vi "Update Ctrls.vi"(8 "error in (no error)":errorcluster, 10 "Columns (All)":string[](array[string]), 11 "Basic Form in":refnum<class "Basic Form.lvclass">) -> (0 "error out":errorcluster, 3 "Basic Form out":refnum<class "Basic Form.lvclass">)   [LabVIEW 2020, in "Form.lvlib" / "Basic Form.lvclass"]
uses:
  Basic Form.lvclass
  C:/Users/User/Desktop/Raman Program/Database OOP/source/Database OOP/Table Libraries/Basic Table/Basic Table Class/Basic Table.lvclass
  Basic Table/Basic Table Class/Basic Table.lvclass/Basic Table.ctl
  Basic Form.lvclass/Basic Form.ctl
  Column Libraries/Field Interfaces/Field Interface Class/Field Interface.lvclass
  C:/Users/User/Desktop/Raman Program/Database OOP/source/Database OOP/Column Libraries/Column Interface/Column Interface Class/Column Interface.lvclass
  Column Libraries/Column Interface/Column Interface Class/Column Interface.lvclass
  Basic Table/Basic Table Class/Basic Table.lvclass
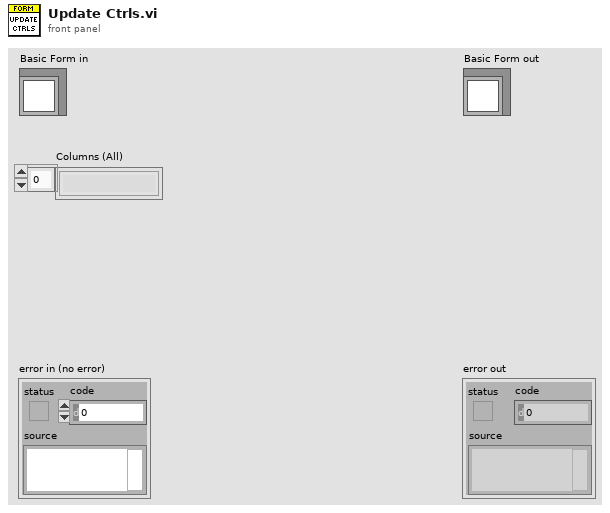
[diagram p1: front panel]
types:
  T1 = map{string, refnum<class "Column Interface.lvclass">}
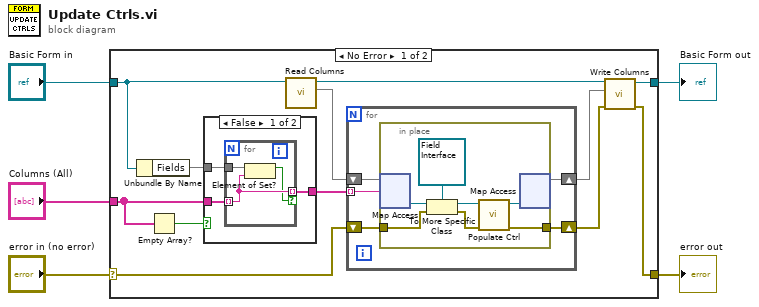
[diagram p0: block diagram]
diagram:
  n1 = case shown="No Error" "error in (no error)" {
    selector: "error in (no error)" -> [w10 w40]
    tunnel: [w6 w40] -> w4
    tunnel: [w8 w39] -> w2
    tunnel: "Basic Form in" -> [w14 w39]
    tunnel: "Columns (All)" -> [w15 _]
    frame No Error {
      n2 = Unbundle By Name(w14) -> ("Fields"=w16:set{string})
      n3 = Empty Array?(array=w15) -> (empty?=w17:bool)
      n4 = case shown="False" w17 {
        tunnel: w16 -> [w31 w37]
        tunnel: [w30 w36] -> w13
        tunnel: w15 -> [w32 _]
        frame False {
          n5 = for {
            tunnel: w32 -> [w34] mode=indexing
            tunnel: w31 -> [w35]
            tunnel: [w34] -> w30 mode=indexing if=w33
            n6 = Element of Set?(10:w34, 11:w35) -> (3:w33:bool)
          }
        }
        frame True {
          n7 = for {
            tunnel: w37 -> [w38] mode=indexing
            tunnel: [w38] -> w36 mode=indexing
          }
        }
      }
      n8 = call "Read Columns.vi"("Basic Table in"=w14) -> ("Columns"=w12:T1, "Basic Table out"=w11:refnum<class "Basic Form.lvclass">)  [unwired: 8 in, 1 out]
      n9 = for {
        tunnel: w13 -> [w22] mode=indexing
        shift-right: [w21] -> w9
        shift-left: w12 -> [w20]
        shift-right: [w19] -> w7
        shift-left: w10 -> [w18]
        n10 = in-place {
          in-place-border: [w24] -> w19
          in-place-border: w18 -> [w23]
          n11 = in-place-map #1(w20, w22) -> (w29:refnum<class "Column Interface.lvclass">)  [unwired: 1 in, 1 out]
          n12 = To More Specific Class(target class=refnum<class "Field Interface.lvclass"> refnum ("Field Interfaces.lvlib:Field Interface.lvclass"), reference=w29, error in=w23) -> (specific class reference=w27:refnum<class "Field Interface.lvclass">, error out=w25:errorcluster)
          n13 = call-dynamic "Populate Ctrl.vi"("error in (no error)"=w25, "Field Interface in"=w27) -> ("error out"=w24:errorcluster, "Field Interface out"=w26:refnum<class "Field Interface.lvclass">)  [unwired: 8 in]
          n14 = in-place-map #1(w26) -> (w21:T1)  [unwired: 1 in, 2 out]
        }
      }
      n15 = call "Write Columns.vi"("error in (no error)"=w7, "Columns"=w9, "Basic Table in"=w11) -> ("error out"=w6:errorcluster, "Basic Table out"=w8:refnum<class "Basic Form.lvclass">)  [unwired: 7 in]
    }
    frame Error {
    }
  }
  "error out" <- w4
  "Basic Form out" <- w2
